vi "Construct Voltage.vi"(8 "error in (no error)":errorcluster, 9 "Slew":dbl, 10 "Voltage":dbl, 11 "VISA resource name":refnum<visa-resource-name>) -> (0 "error out":errorcluster, 3 "VISA resource name out":refnum<visa-resource-name>)   [LabVIEW 2019, in "79XRP.lvlib" / "79XRP.lvclass"]
uses:
  Library/79XRP.lvclass
  <instrlib>/Keysight RP7900 Series/Keysight RP7900 Series.lvlib
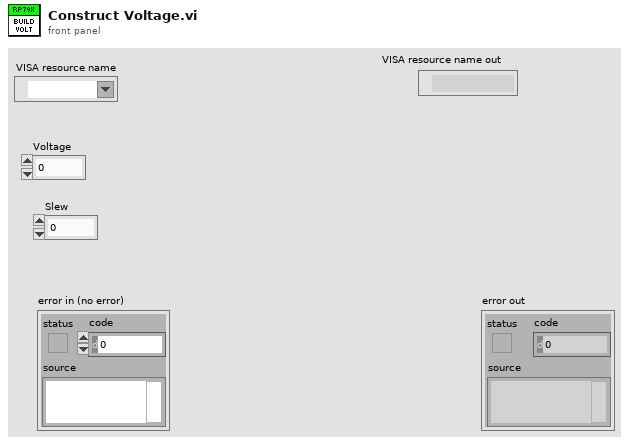
[diagram p1: front panel]
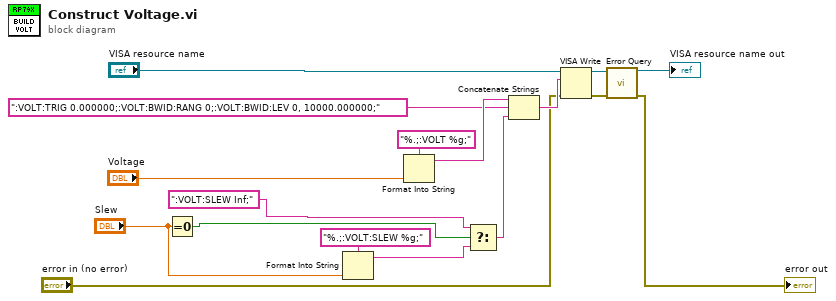
[diagram p0: block diagram]
diagram:
  n1 = Equal To 0?(x="Slew") -> (x = 0?=w2:bool)
  n2 = Format Into String(format string="%.;:VOLT:SLEW %g;", "Slew") -> (resulting string=w4:string)  [unwired: 2 in, 1 out]
  n3 = Format Into String(format string="%.;:VOLT %g;", "Voltage") -> (resulting string=w10:string)  [unwired: 2 in, 1 out]
  n4 = Select(t=":VOLT:SLEW Inf;" ("format string"), s=w2, f=w4) -> (s? t:f=w5:string)
  n5 = Concatenate Strings(w10, ":VOLT:TRIG 0.000000;:VOLT:BWID:RANG 0;:VOLT:BWID:LEV 0, 10000.000000;" ("string"), w5) -> (w11:string)
  n6 = VISA Write(VISA resource name="VISA resource name", write buffer=w11, error in (no error)="error in (no error)") -> (VISA resource name out=w15:refnum<visa-resource-name>, error out=w16:errorcluster)  [unwired: 1 out]
  n7 = call <instrlib>:"Error Query.vi"("error in (no error)"=w16, "VISA resource name"=w15) -> ("error out"=→"error out":errorcluster, "VISA resource name out"=→"VISA resource name out":refnum<visa-resource-name>)  [unwired: 6 in, 2 out]
